vi "log_main.vi"(7 "FGV_mods":T1, 8 "Error In":errorcluster, 11 "DataIn":variant) -> (0 "Error Out":errorcluster, 3 "DataOut":variant)   [LabVIEW 2016]
uses:
  log_mods.ctl
  log_data.ctl
  log_status.ctl
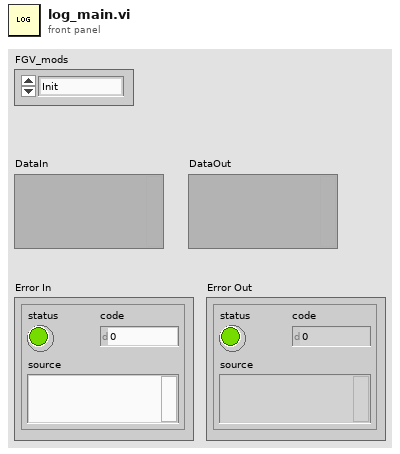
[diagram p1: front panel]
types:
  T1 = typedef "log_mods.ctl" = enum16{"Init", "LogFileRefnum", "SetStatus", "WriteAcel", "WriteToLog", "End"}
  T2 = typedef "log_data.ctl" = cluster{"log_status":T3, "Acel_data":dbl[], "LogRef":refnum<vi>, "log_file":refnum<file>}
  T3 = typedef "log_status.ctl" = enum16{"Init", "Ready", "Config", "Running", "Error", "End"}
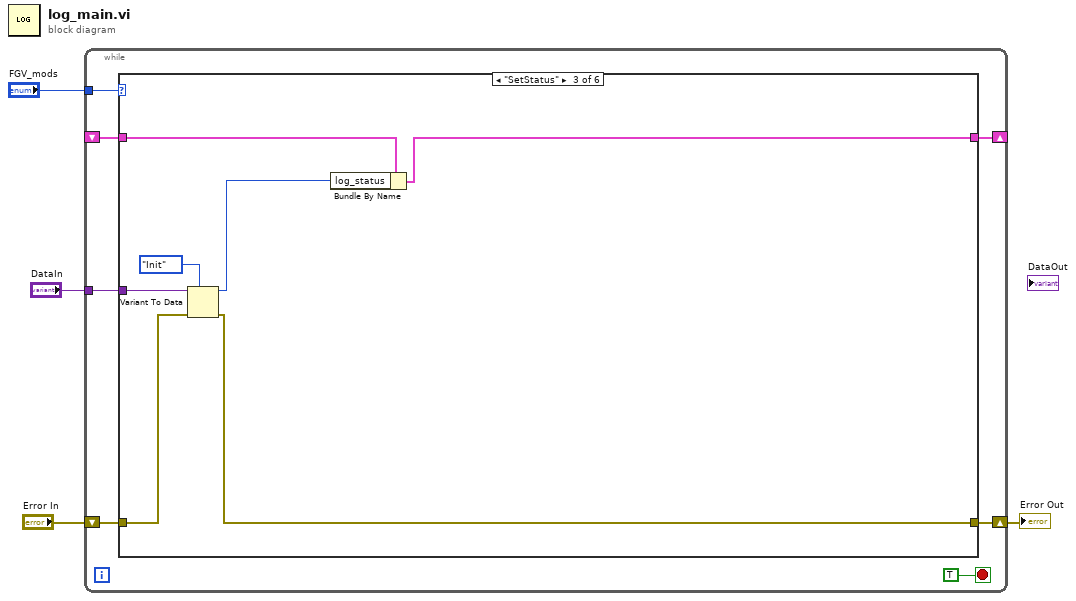
[diagram p0: block diagram]
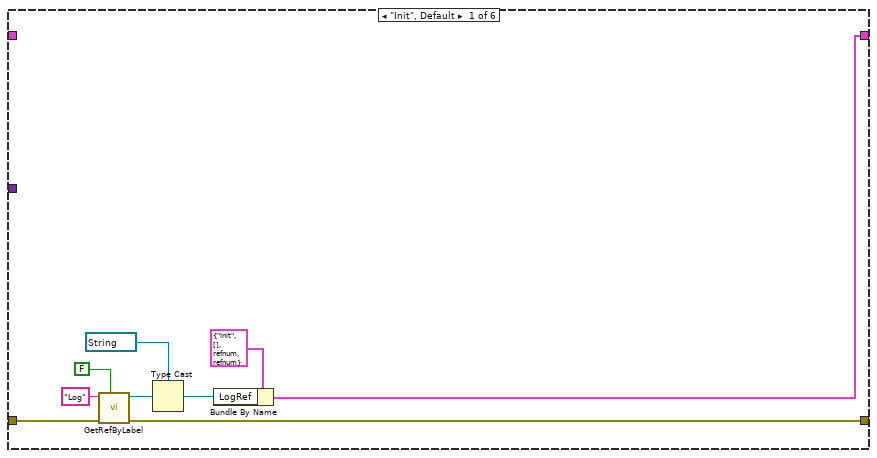
[diagram p2: hidden frame]
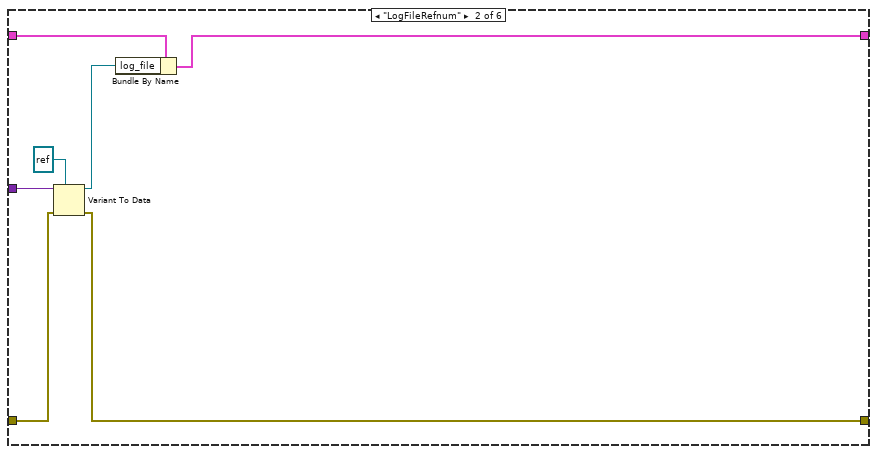
[diagram p3: hidden frame]
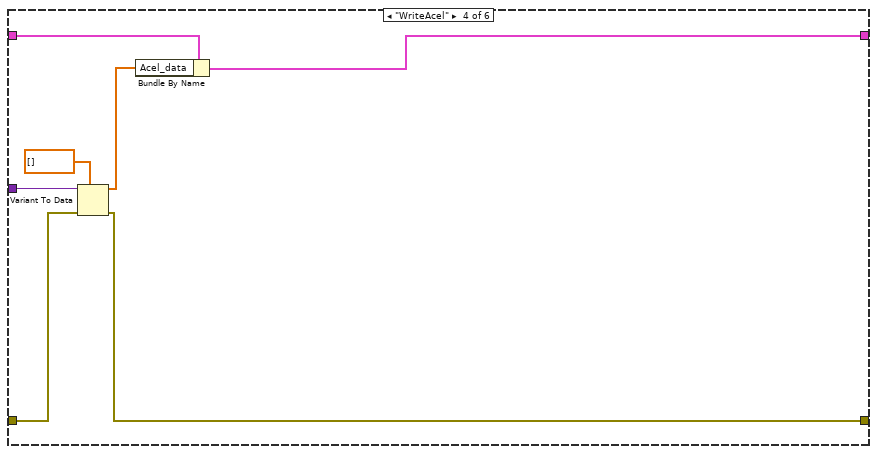
[diagram p4: hidden frame]
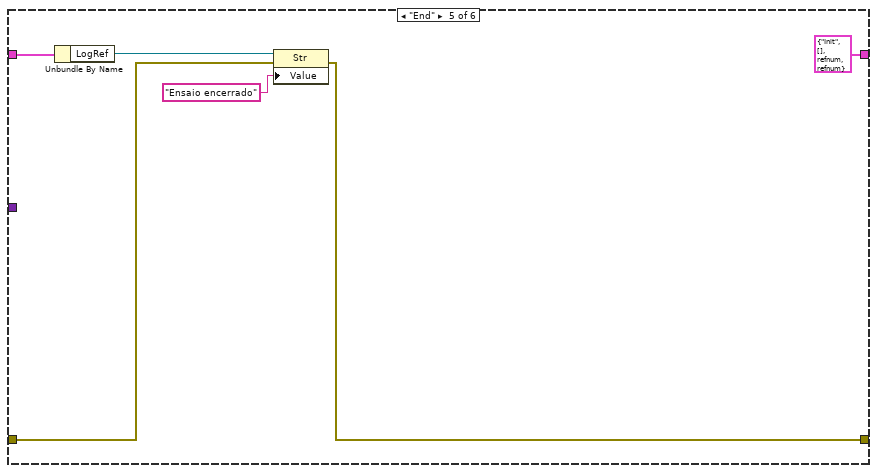
[diagram p5: hidden frame]
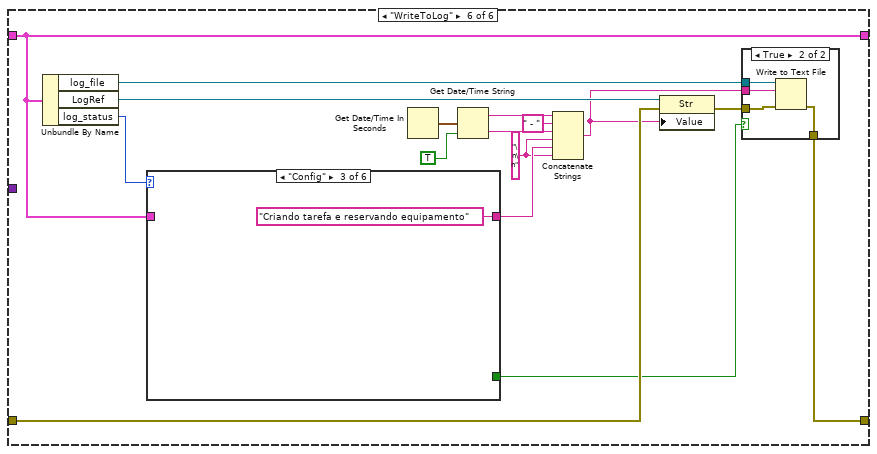
[diagram p6: hidden frame]
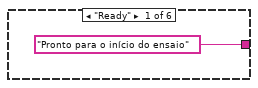
[diagram p8: hidden frame]
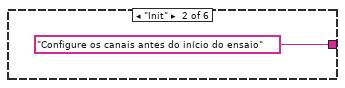
[diagram p9: hidden frame]
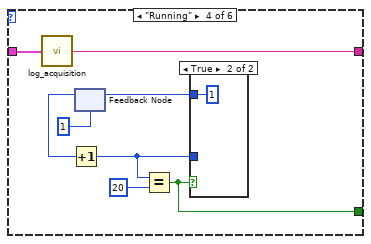
[diagram p10: hidden frame]
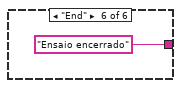
[diagram p13: hidden frame]
diagram:
  n1 = while {
    tunnel: "DataIn" -> [w10]
    tunnel: "FGV_mods" -> [w9]
    shift-right: [w8] -> _
    shift-left: _ -> [w7]
    shift-right: [w5] -> w1
    shift-left: "Error In" -> [w6]
    stop <- TRUE stop-if-true
    n2 = case shown="\"SetStatus\"" w9 {
      tunnel: w10 -> [_ w26 w32 w39 _ _]
      tunnel: [w13 w21 w33 w40 T2 {"log_status"=enum."Init", "Acel_data"=[], "LogRef"=refnum, "log_file"=refnum} ("log_data") w62] -> w8
      tunnel: w7 -> [_ w23 w34 w41 w46 w62]
      tunnel: w6 -> [w18 w25 w31 w38 w43 w60]
      tunnel: [w12 w24 w28 w37 w42 w49] -> w5
      frame "Init", Default {
        n3 = call "GetRefByLabel.vi"("InsideTab"=FALSE, "error in"=w18, "Label"="Log") -> ("error out"=w12:errorcluster, "Ctl Refnum"=w17:refnum<vi>)  [unwired: 6 in, 1 out]
        n4 = Type Cast(type=refnum<vi> refnum ("Log"), x=w17) -> (*(type *) &x=w14:refnum<vi>)
        n5 = Bundle By Name(cluster=T2 {"log_status"=enum."Init", "Acel_data"=[], "LogRef"=refnum, "log_file"=refnum} ("log_data"), "LogRef"=w14) -> (w13:T2)
      }
      frame "LogFileRefnum" {
        n6 = Variant To Data(error in=w25, type=refnum<file> refnum ("log_file"), Variant=w26) -> (data=w22:refnum<file>, error out=w24:errorcluster)
        n7 = Bundle By Name(cluster=w23, "log_file"=w22) -> (w21:T2)
      }
      frame "SetStatus" {
        n8 = Variant To Data(error in=w31, type=log_status."Init" ("log_status"), Variant=w32) -> (data=w29:T3, error out=w28:errorcluster)
        n9 = Bundle By Name(cluster=w34, "log_status"=w29) -> (w33:T2)
      }
      frame "WriteAcel" {
        n10 = Variant To Data(error in=w38, type=dbl[] [] ("SG_data"), Variant=w39) -> (data=w35:dbl[], error out=w37:errorcluster)
        n11 = Bundle By Name(cluster=w41, "Acel_data"=w35) -> (w40:T2)
      }
      frame "End" {
        n12 = Unbundle By Name(w46) -> ("LogRef"=w45:refnum<vi>)
        n13 = property class="Str"(reference=w45, error in=w43, "Value"="Ensaio encerrado") -> (error out=w42:errorcluster)  [unwired: 1 out]
      }
      frame "WriteToLog" {
        w48 = "\n\n" ("string")
        n14 = Unbundle By Name(w62) -> ("log_file"=w51:refnum<file>, "LogRef"=w61:refnum<vi>, "log_status"=w63:T3)
        n15 = case shown="\"Config\"" w63 {
          tunnel: w62 -> [_ _ _ w79 _ _]
          tunnel: ["Pronto para o início do ensaio" ("Value") "Configure os canais antes do início do ensaio" ("Value") "Criando tarefa e reservando equipamento" ("Value") w78 _ "Ensaio encerrado" ("Value")] -> w55
          tunnel: [_ _ _ w72 _ _] -> w53
          frame "Ready" {
          }
          frame "Init" {
          }
          frame "Config" {
          }
          frame "Running" {
            n16 = call "log_acquisition.vi"("log_data"=w79) -> ("Log"=w78:string)
            n17 = feedback #1(1) -> (w77:i32)
            n18 = Increment(x=w77) -> (x+1=w73:i32)
            n19 = Equal?(x=w73, y=20) -> (x = y?=w72:bool)
            n20 = case shown="True" w72 {
              tunnel: [w80 1 ("y")] -> w74
              tunnel: w73 -> [w80 _]
              frame False {
              }
              frame True {
              }
            }
            n21 = feedback-in #1(w74) -> ()
          }
          frame "Error" {
          }
          frame "End" {
          }
        }
        n22 = Get Date/Time In Seconds() -> (seconds since 1Jan1904=w59:timestamp)
        n23 = Get Date/Time String(seconds (now)=w59, want seconds? (F)=TRUE) -> (date string=w58:string, time string=w57:string)  [unwired: 1 in]
        n24 = Concatenate Strings(w58, " - " ("string"), w57, w48, w55, w48) -> (w50:string)
        n25 = property class="Str"(reference=w61, error in=w60, "Value"=w50) -> (error out=w52:errorcluster)  [unwired: 1 out]
        n26 = case shown="True" w53 {
          tunnel: w52 -> [w64 w68]
          tunnel: w51 -> [_ w67]
          tunnel: w50 -> [_ w66]
          tunnel: [w64 w65] -> w49
          frame False {
          }
          frame True {
            n27 = Write to Text File(file (use dialog)=w67, text=w66, error in=w68) -> (error out=w65:errorcluster)  [unwired: 1 in, 2 out]
          }
        }
      }
    }
  }
  "Error Out" <- w1
